vi "多参数传感器参数读取.vi"(8 "Error in":errorcluster caption="Error in (no error)") -> (0 "error out":errorcluster, 2 "modbus":u16[](array[numeric]), 3 "添加的数组":string[][](array[string]))   [LabVIEW 2016, in "斯坦道原位多参数.lvlib"]
panel:
  in  "下拉列表":u16(ring) items=["氨氮"=3, "水温"=9, "pH"=10, "溶解氧"=11, "电导率"=12, "浊度"=13, "叶绿素a"=14, "藻密度"=15, "蓝绿藻"=16, "氧化还原电位"=17, "溶解氧%"=18, "盐度"=19, "水中油"=20, "高锰酸盐指数"=21, "化学需氧量"=22, "比电导率"=23, "总溶解固体"=24, "pH电极电位"=25]
  in  "传感器区":i32(listbox)
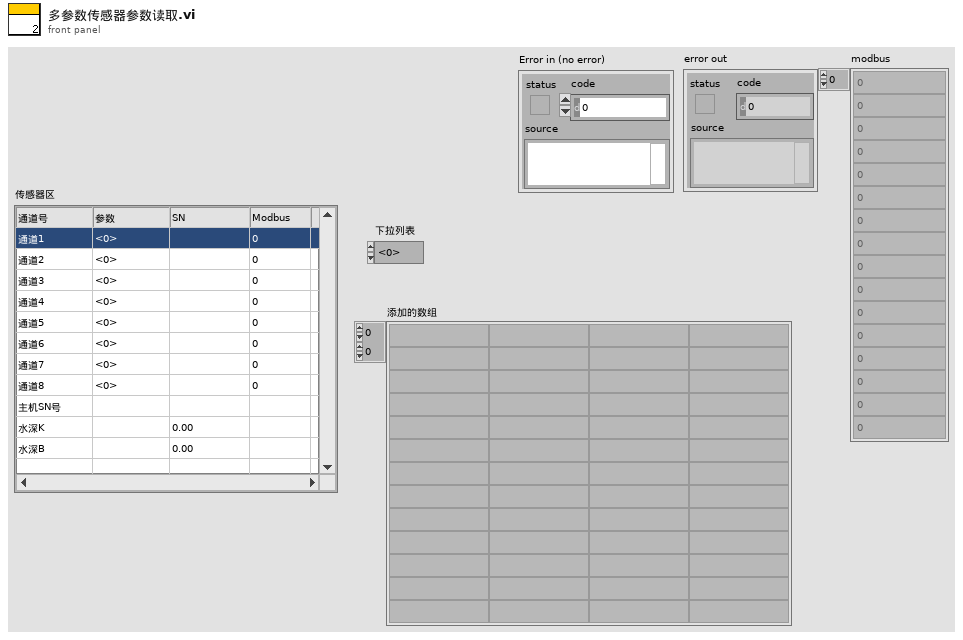
[diagram p1: front panel]
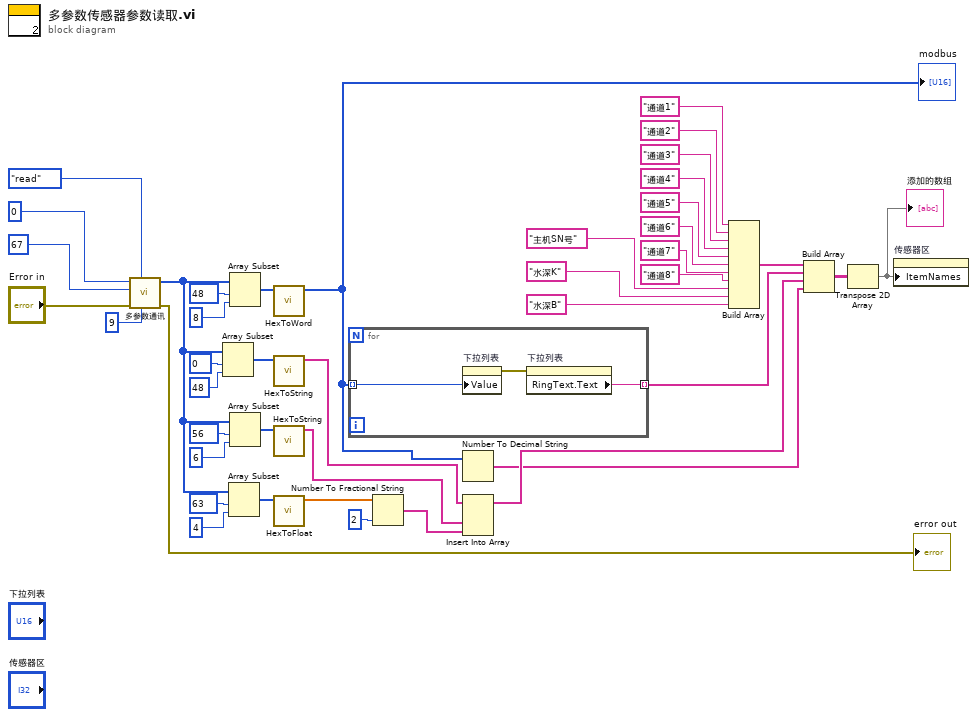
[diagram p0: block diagram]
diagram:
  n1 = call "多参数通讯.vi"("Slave ID"=u8 9, "STEP"=enum16{"open", "read", "write", "close"}."read", "Error in"="Error in", "quantity"=u16 67, "starting address"=u16 0) -> ("error out"=→"error out":errorcluster, "Registers"=w1:u16[])  [unwired: 4 in, 1 out]
  n2 = Array Subset(array=w1, index=u16 0 ("starting address"), length=48 ("长度")) -> (w8:u16[])
  n3 = Array Subset(array=w1, index=u16 63 ("starting address"), length=4 ("长度")) -> (w4:u16[])
  n4 = Array Subset(array=w1, index=u16 48 ("starting address"), length=8 ("长度")) -> (w25:u16[])
  n5 = Array Subset(array=w1, index=u16 56 ("starting address"), length=6 ("长度")) -> (w23:u16[])
  n6 = call "HexToWord.vi"("数组"=w25) -> ("WORD"=w15:u16[])  [unwired: 10 in]
  "modbus" <- w15
  n7 = call "HexToString.vi"("数组"=w8) -> ("STRING"=w22:string[])  [unwired: 10 in]
  n8 = call "HexToString.vi"("数组"=w23) -> ("STRING"=w21:string[])  [unwired: 10 in]
  n9 = call "HexToFloat.vi"("数组"=w4) -> ("FLOAT"=w3:sgl[])  [unwired: 10 in]
  n10 = for {
    tunnel: w15 -> [w44] mode=indexing
    tunnel: [w43] -> w27 mode=indexing
    n11 = property on="下拉列表" class="Ring (strict)"("Value"=w44) -> (error out=w45:errorcluster)  [unwired: 2 in, 1 out]
    n12 = property on="下拉列表" class="Ring (strict)"(error in=w45) -> ("RingText.Text"=w43:string)  [unwired: 1 in, 2 out]
  }
  n13 = Number To Fractional String(number=w3, precision (6)=i16 2 ("精度(6)")) -> (F-format string=w20:string[])  [unwired: 2 in]
  n14 = Number To Decimal String(number=w15) -> (decimal integer string=w14:string[])  [unwired: 1 in]
  n15 = Insert Into Array(array=w22, new element #1=w21, new element #2=w20) -> (w19:string[])  [unwired: 1 in]
  n16 = Build Array("通道1", "通道2", "通道3", "通道4", "通道5", "通道6", "通道7", "通道8", "主机SN号", "水深K", "水深B") -> (w32:string[])
  n17 = Build Array(w32, w27, w19, w14) -> (w31:string[][])
  n18 = Transpose 2D Array(2D array=w31) -> (transposed array=w13:string[][])
  "添加的数组" <- w13
  n19 = property on="传感器区" class="MCListbox (strict)"("ItemNames"=w13) -> ()  [unwired: 2 in, 2 out]
